vi "ex2.vi"() -> ()   [LabVIEW 2019]
panel:
  out "Array":bool[](array[boolean])
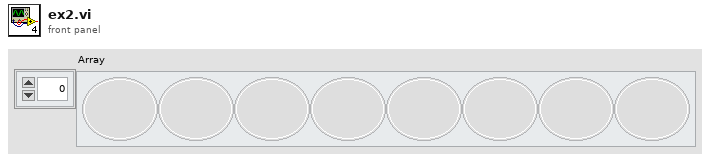
[diagram p1: front panel]
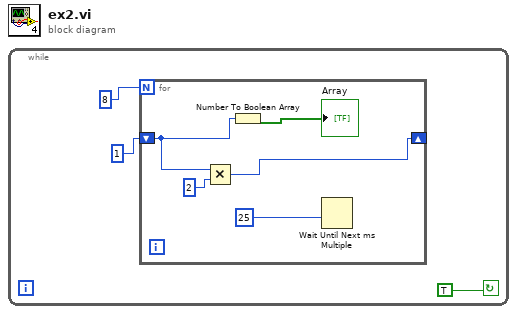
[diagram p0: block diagram]
diagram:
  n1 = while {
    stop <- TRUE continue-if-true
    n2 = for {
      N: 8 -> [_]
      shift-right: [w4] -> _
      shift-left: 1 -> [w5]
      n3 = Multiply(x=w5, y=2) -> (x*y=w4:i32)
      n4 = Number To Boolean Array(number=w5) -> (Boolean array=→"Array":bool[])
      n5 = Wait Until Next ms Multiple(millisecond multiple=25) -> ()  [unwired: 1 out]
    }
  }
